vi "tap.vi"(5 "COM Bluegiga in":refnum<visa-resource-name>, 9 "error in (no error)":errorcluster) -> (1 "error out":errorcluster, 3 "COM Bluegiga out":refnum<visa-resource-name>, 4 "X UP":bool, 6 "X DOWN":bool, 8 "Count":u8, 10 "Y UP":bool, 12 "Z UP":bool, 13 "Z DOWN":bool, 15 "Y DOWN":bool)   [LabVIEW 2020]
panel:
  out "characteristic value":u8[](array[numeric])
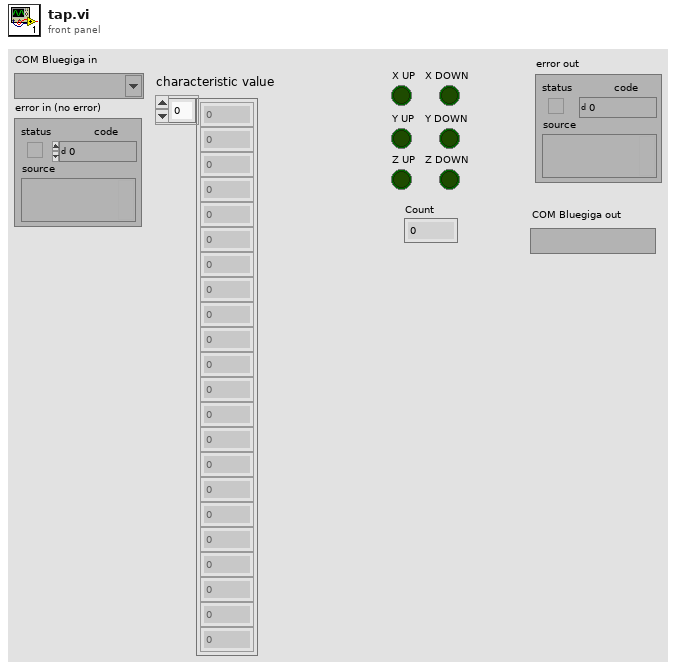
[diagram p1: front panel]
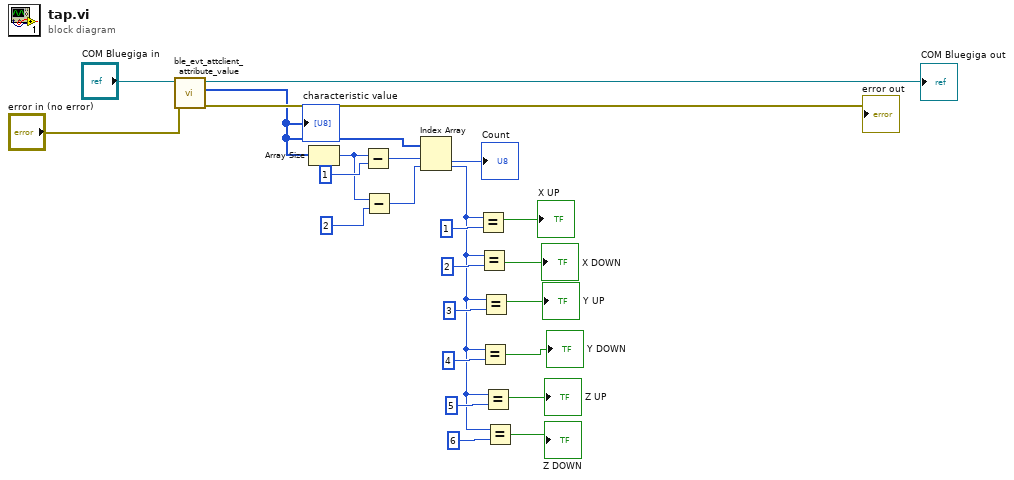
[diagram p0: block diagram]
diagram:
  n1 = call <vilib>:"ble_evt_attclient_attribute_value.vi"("error in (no error)"="error in (no error)", "COM Bluegiga in"="COM Bluegiga in") -> ("error out"=→"error out":errorcluster, "characteristic value"=w20:u8[], "COM Bluegiga out"=→"COM Bluegiga out":refnum<visa-resource-name>)  [unwired: 6 in, 1 out]
  "characteristic value" <- w20
  n2 = Array Size(array=w20) -> (size(s)=w15:i32)
  n3 = Subtract(x=w15, y=1) -> (x-y=w21:i32)
  n4 = Subtract(x=w15, y=2) -> (x-y=w14:i32)
  n5 = Index Array(array=w20, index #1=w21, index #2=w14) -> (element #1=→"Count":u8, element #2=w1:u8)
  n6 = Equal?(x=w1, y=u8 1) -> (x = y?=→"X UP":bool)
  n7 = Equal?(x=w1, y=u8 2) -> (x = y?=→"X DOWN":bool)
  n8 = Equal?(x=w1, y=u8 4) -> (x = y?=→"Y DOWN":bool)
  n9 = Equal?(x=w1, y=u8 3) -> (x = y?=→"Y UP":bool)
  n10 = Equal?(x=w1, y=u8 5) -> (x = y?=→"Z UP":bool)
  n11 = Equal?(x=w1, y=u8 6) -> (x = y?=→"Z DOWN":bool)
